vi "Oscilloscope_General_Settings.vi"() -> ()   [LabVIEW 2020]
uses:
  Return_To_Interface.ctl
panel:
  in  "Return to Interface":T1
  # "PER ANDREA: FARE ANCHE UN ALTRO VI D UTILIZZARE NELLA FLAT SEQUENCE INIZIALE, DOVE SI DA' IL \nBENVENUTO ALL'UTENTE DICENDO LE CARATTERISTICHE DELLO STRUMENTO E IL NOME DELLA MIA TESI\nCON TUTTE LE FRASI INIZIALI. QUESTO E' IL PRIMO APPROCCIO CHE DEVE AVERE L'UTENTE CON IL\nPROGRAMMA PERCIO DEVE ESSERE ACCATTIVANTE, POI SI ANDRANNO AD IMPOSTARE LE PRIME \nIMPOSTAZIONI INIZIALI. DA QUESTO PRIMO ELEMENTO POTREBBE ESSERCI UNA SPECIE DI MENU\nPRELIMINARE, DOVE IMPOSTIAMO I SETTAGGI INIZIALI PER POI ANDARE NEL PROGRAMMA VERO E PROPRIO \nDELL'OSCILLOSCOPIO."
  # "QUI CI VUOLE UN MESSAGGIO DOVE SPIEGA COME SI SETTANO LE IMPOSTAZIONI DELLO STRUMENTO E COME FUNZIONA\nLA PULSANTIERA CHE CI SARA IN QUESTO PUNTO. DEVO PROVARE A SIMULARE IN TUTTO E PER TUTTO LA PULSANTIERA \nDELL'OSCILLOSCOPIO E TENERE QUESTO VI PER I SETTAGGI"
  # "OSCILLOSCOPE SETTINGS"
  # "Qui voglio gestire le impostazioni\ndell'oscilloscopio e alla pressione del tasto FATTO\nvado al programma dell'interfaccia dell'oscilloscopio,\ndove posso fare il resto.\n\nQuesta è una pulsantiera!"
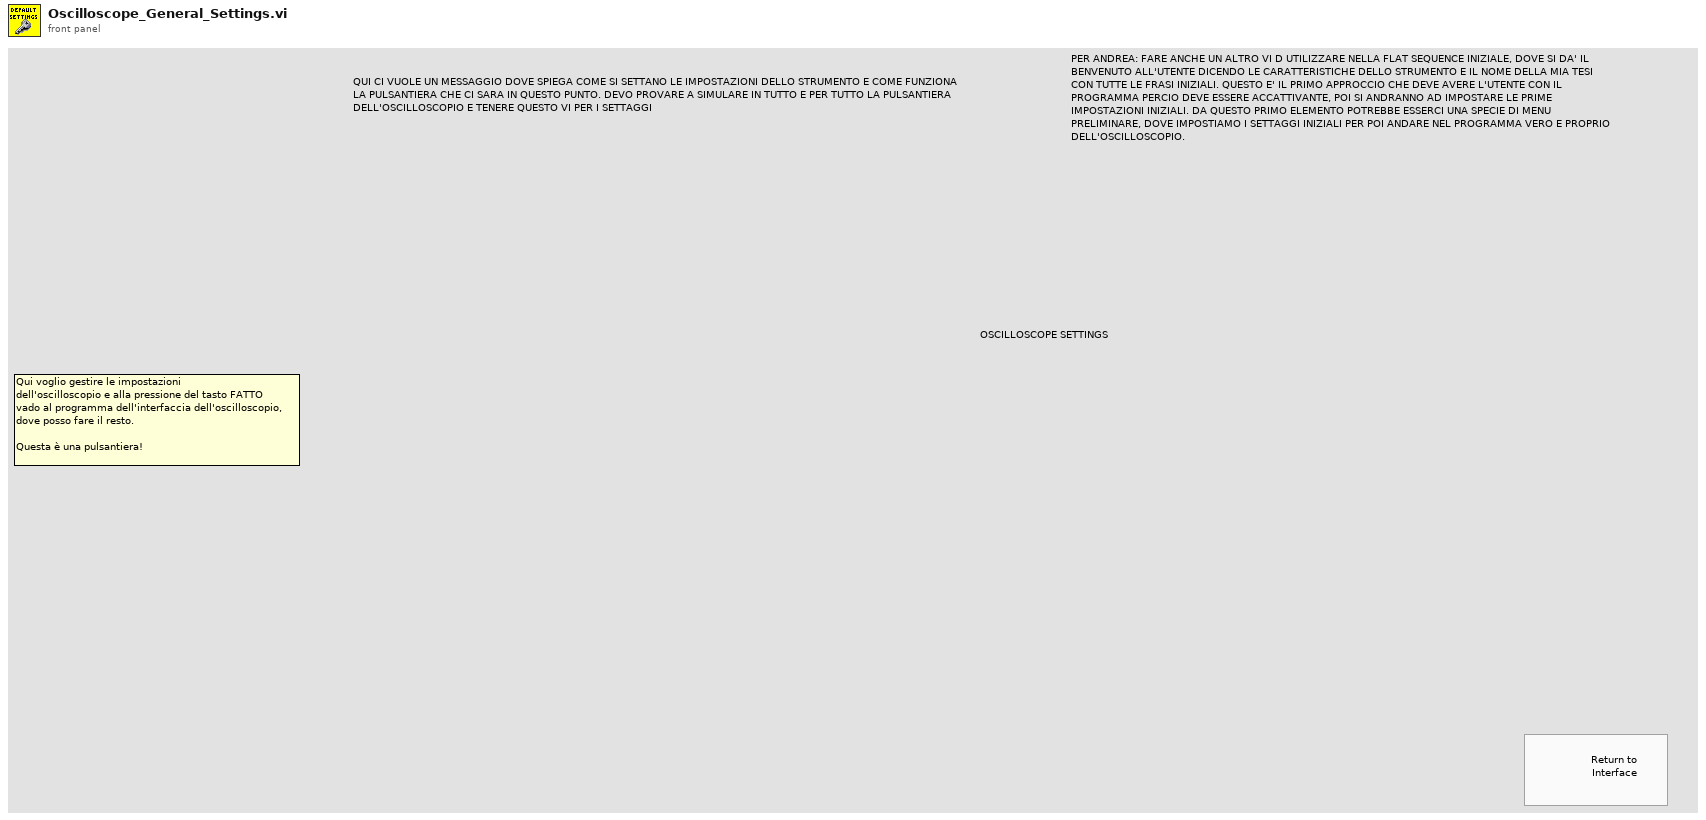
[diagram p1: front panel]
types:
  T1 = typedef "Return_To_Interface.ctl" = bool
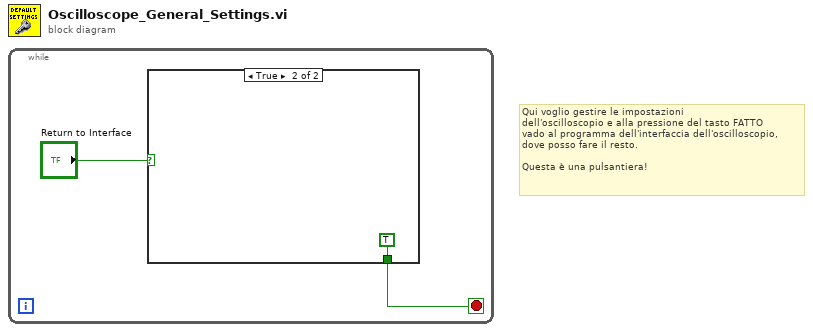
[diagram p0: block diagram]
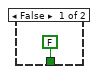
[diagram p2: hidden frame]
diagram:
  # "Qui voglio gestire le impostazioni\ndell'oscilloscopio e alla pressione del tasto FATTO\nvado al programma dell'interfaccia dell'oscilloscopio,\ndove posso fare il resto.\n\nQuesta è una pulsantiera!"
  n1 = while {
    stop <- w2 stop-if-true
    n2 = case shown="True" "Return to Interface" {
      tunnel: [FALSE TRUE] -> w2
      frame False {
      }
      frame True {
      }
    }
  }
